vi "SNMP Byte Array to Int32.vi"(0 "DataArray":u8[](array[numeric]) format="%.0x") -> (1 "Unsigned Value":u32, 2 "Signed Value":i32)   [LabVIEW 2017]
doc: "This VI is used to convert a byte array representation of a number into a single numeric value. The VI outputs the numeric value as both a signed (INT 32) and an unsigned (UINT 32) value."
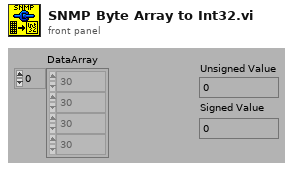
[diagram p1: front panel]
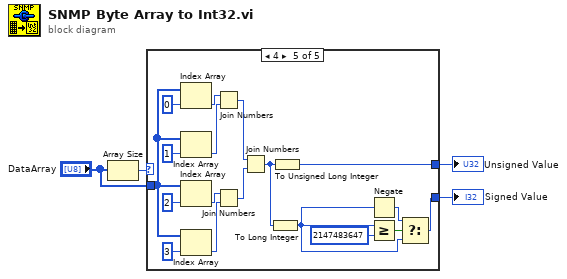
[diagram p0: block diagram]
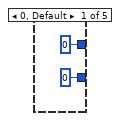
[diagram p2: hidden frame]
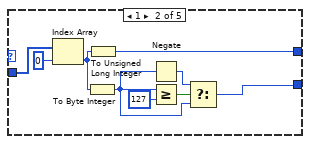
[diagram p3: hidden frame]
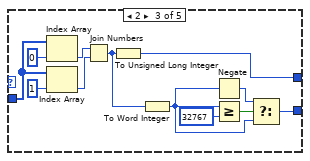
[diagram p4: hidden frame]
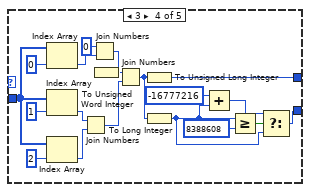
[diagram p5: hidden frame]
diagram:
  n1 = Array Size(array="DataArray") -> (size(s)=w4:i32)
  n2 = case shown="4" w4 {
    tunnel: "DataArray" -> [_ w15 w25 w43 w56]
    tunnel: [u32 0 w13 w22 w36 w53] -> w2
    tunnel: [0 w7 w17 w32 w47] -> w1
    frame 0, Default {
    }
    frame 1 {
      n3 = Index Array(array=w15, index=0) -> (element=w9:u8)
      n4 = To Byte Integer(number=w9) -> (8bit integer=w8:i8)
      n5 = To Unsigned Long Integer(number=w9) -> (unsigned 32bit integer=w13:u32)
      n6 = Negate(x=w8) -> (-x=w10:i8)
      n7 = Greater Or Equal?(x=w8, y=i8 127) -> (x >= y?=w11:bool)
      n8 = Select(t=w10, s=w11, f=w8) -> (s? t:f=w7:i8)
    }
    frame 2 {
      n9 = Index Array(array=w25, index=0) -> (element=w24:u8)
      n10 = Index Array(array=w25, index=1) -> (element=w23:u8)
      n11 = Join Numbers(hi=w24, lo=w23) -> ((hi.lo)=w16:u16)
      n12 = To Unsigned Long Integer(number=w16) -> (unsigned 32bit integer=w22:u32)
      n13 = To Word Integer(number=w16) -> (16bit integer=w21:i16)
      n14 = Negate(x=w21) -> (-x=w20:i16)
      n15 = Greater Or Equal?(x=w21, y=i16 32767) -> (x >= y?=w19:bool)
      n16 = Select(t=w20, s=w19, f=w21) -> (s? t:f=w17:i16)
    }
    frame 3 {
      n17 = Index Array(array=w43, index=0) -> (element=w37:u8)
      n18 = Index Array(array=w43, index=1) -> (element=w40:u8)
      n19 = Index Array(array=w43, index=2) -> (element=w41:u8)
      n20 = Join Numbers(hi=w40, lo=w41) -> ((hi.lo)=w39:u16)
      n21 = Join Numbers(hi=u16 0, lo=w37) -> ((hi.lo)=w42:u32)
      n22 = To Unsigned Word Integer(number=w42) -> (unsigned 16bit integer=w28:u16)
      n23 = Join Numbers(hi=w28, lo=w39) -> ((hi.lo)=w33:u32)
      n24 = To Unsigned Long Integer(number=w33) -> (unsigned 32bit integer=w36:u32)
      n25 = To Long Integer(number=w33) -> (32bit integer=w30:i32)
      n26 = Add(x=-16777216, y=w30) -> (x+y=w29:i32)
      n27 = Greater Or Equal?(x=w30, y=8388608) -> (x >= y?=w35:bool)
      n28 = Select(t=w29, s=w35, f=w30) -> (s? t:f=w32:i32)
    }
    frame 4 {
      n29 = Index Array(array=w56, index=0) -> (element=w63:u8)
      n30 = Index Array(array=w56, index=1) -> (element=w64:u8)
      n31 = Index Array(array=w56, index=2) -> (element=w58:u8)
      n32 = Index Array(array=w56, index=3) -> (element=w57:u8)
      n33 = Join Numbers(hi=w63, lo=w64) -> ((hi.lo)=w55:u16)
      n34 = Join Numbers(hi=w58, lo=w57) -> ((hi.lo)=w54:u16)
      n35 = Join Numbers(hi=w55, lo=w54) -> ((hi.lo)=w48:u32)
      n36 = To Long Integer(number=w48) -> (32bit integer=w49:i32)
      n37 = To Unsigned Long Integer(number=w48) -> (unsigned 32bit integer=w53:u32)
      n38 = Negate(x=w49) -> (-x=w50:i32)
      n39 = Greater Or Equal?(x=w49, y=2147483647) -> (x >= y?=w51:bool)
      n40 = Select(t=w50, s=w51, f=w49) -> (s? t:f=w47:i32)
    }
  }
  "Unsigned Value" <- w2
  "Signed Value" <- w1
